vi "EC_DC_relay_control_subVI.vi"(10 "BoardNum":u32=1, 11 "Enum":T1(ring)) -> ()   [LabVIEW 2021]
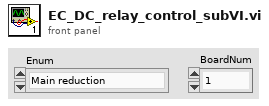
[diagram p1: front panel]
types:
  T1 = enum16{"Main reduction", "Reverse reduction", "Turn off all DC"}
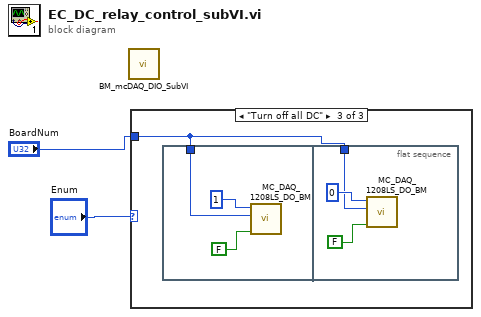
[diagram p0: block diagram]
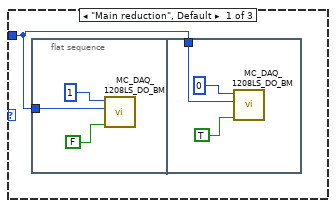
[diagram p2: hidden frame]
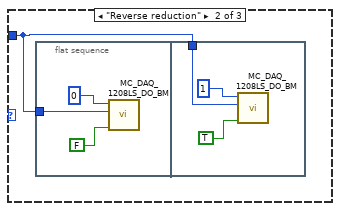
[diagram p3: hidden frame]
diagram:
  n1 = call "BM_mcDAQ_DIO_SubVI.vi"() -> ()  [unwired: 11 in, 1 out]
  n2 = case shown="\"Turn off all DC\"" "Enum" {
    tunnel: "BoardNum" -> [w3 w10 w17]
    frame "Main reduction", Default {
      n3 = flat-sequence {
        tunnel: w3 -> [w4]
        tunnel: w3 -> [w7]
        frame #0 {
          n4 = call "MC_DAQ_1208LS_DO_BM.vi"("BitValue"=FALSE, "BoardNum"=w4, "BitNum"=u32 1) -> ()  [unwired: 8 in, 1 out]
        }
        frame #1 {
          n5 = call "MC_DAQ_1208LS_DO_BM.vi"("BitValue"=TRUE, "BoardNum"=w7, "BitNum"=u32 0) -> ()  [unwired: 8 in, 1 out]
        }
      }
    }
    frame "Reverse reduction" {
      n6 = flat-sequence {
        tunnel: w10 -> [w11]
        tunnel: w10 -> [w14]
        frame #0 {
          n7 = call "MC_DAQ_1208LS_DO_BM.vi"("BitValue"=FALSE, "BoardNum"=w11, "BitNum"=u32 0) -> ()  [unwired: 8 in, 1 out]
        }
        frame #1 {
          n8 = call "MC_DAQ_1208LS_DO_BM.vi"("BitValue"=TRUE, "BoardNum"=w14, "BitNum"=u32 1) -> ()  [unwired: 8 in, 1 out]
        }
      }
    }
    frame "Turn off all DC" {
      n9 = flat-sequence {
        tunnel: w17 -> [w18]
        tunnel: w17 -> [w21]
        frame #0 {
          n10 = call "MC_DAQ_1208LS_DO_BM.vi"("BitValue"=FALSE, "BoardNum"=w18, "BitNum"=u32 1) -> ()  [unwired: 8 in, 1 out]
        }
        frame #1 {
          n11 = call "MC_DAQ_1208LS_DO_BM.vi"("BitValue"=FALSE, "BoardNum"=w21, "BitNum"=u32 0) -> ()  [unwired: 8 in, 1 out]
        }
      }
    }
  }
